vi "QueryServer_Start.vi"(7 "error in (no error)":errorcluster, 8 "Server Key File (.key)":path, 9 "Server Certificate File (.crt)":path, 10 "Server Address":string) -> (0 "error out":errorcluster, 2 "Event Registration Refnum":refnum<event-registration>, 3 "Server Info":T2)   [LabVIEW 2019, in "labview-grpc-query-server.lvlib"]
uses:
  labview-grpc-query-server.lvlib
  QueryServer_InvokeEventData.ctl
  gRPC interface/Server API/typeDefs/grpcId.ctl
  gRPC interface/Server API/typeDefs/Message Metadata.ctl
  gRPC interface/Server API/typeDefs/Message Element Metadata.ctl
  gRPC interface/Server API/typeDefs/Message Element Type.ctl
  gRPC interface/gprc-lvsupport.lvlib
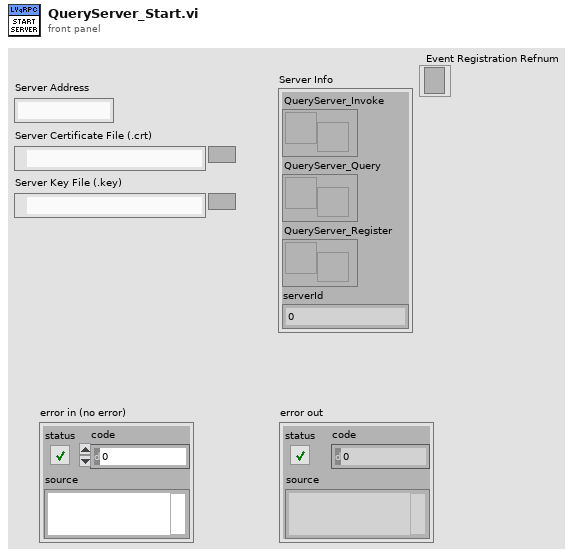
[diagram p1: front panel]
types:
  T1 = typedef "gprc-lvsupport.lvlib/grpcId.ctl" = u64
  T2 = cluster{"QueryServer_Invoke":refnum<user-event>, "QueryServer_Query":refnum<user-event>, "QueryServer_Register":refnum<user-event>, "serverId":T1}
  T3 = typedef "gprc-lvsupport.lvlib/Message Metadata.ctl" = cluster{"Name":string, "Elements":T4[]}
  T4 = typedef "gprc-lvsupport.lvlib/Message Element Metadata.ctl" = cluster{"Embedded Message Name":string, "Protobuf Index":i32, "MessageElementType":T5, "Repeated":bool}
  T5 = typedef "gprc-lvsupport.lvlib/Message Element Type.ctl" = enum32{"Int32Value", "FloatValue", "DoubleValue", "BoolValue", "StringValue", "MessageValue", ""}
  T6 = cluster{"QueryServer_Invoke":refnum<user-event>, "QueryServer_Query":refnum<user-event>, "QueryServer_Register":refnum<user-event>, "gRPCid":T1}
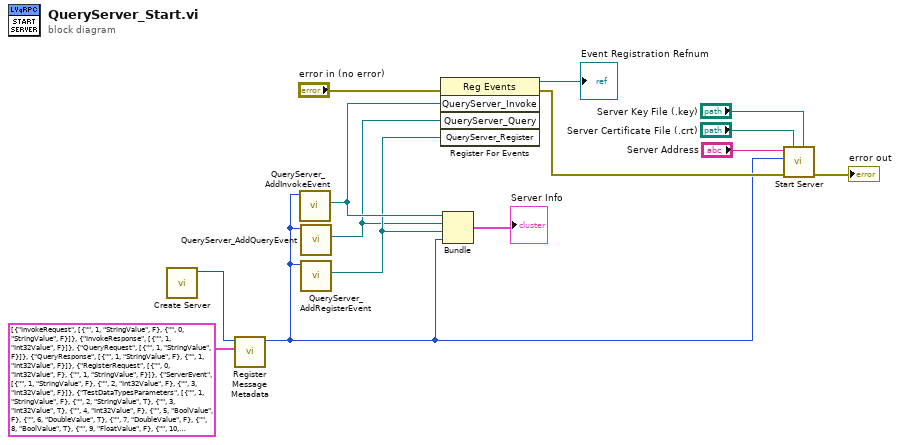
[diagram p0: block diagram]
diagram:
  n1 = call "Create Server.vi"() -> ("gRPCid"=w10:T1)  [unwired: 11 in]
  n2 = call "Register Message Metadata.vi"("Messages"=T3[] [{"Name"="InvokeRequest", "Elements"=[{"Embedded Message Name"="", "Protobuf Index"=1, "MessageElementType"=enum."StringValue", "Repeated"=FALSE}, {"Embedded Message Name"="", "Protobuf Index"=0, "MessageElementType"=enum."StringValue", "Repeated"=FALSE}]}, {"Name"="InvokeResponse", "Elements"=[{"Embedded Message Name"="", "Protobuf Index"=1, "MessageElementType"=enum."Int32Value", "Repeated"=FALSE}]}, {"Name"="QueryRequest", "Elements"=[{"Embedded Message Name"="", "Protobuf Index"=1, "MessageElementType"=enum."StringValue", "Repeated"=FALSE}]}, {"Name"="QueryResponse", "Elements"=[{"Embedded Message Name"="", "Protobuf Index"=1, "MessageElementType"=enum."StringValue", "Repeated"=FALSE}, {"Embedded Message Name"="", "Protobuf Index"=1, "MessageElementType"=enum."Int32Value", "Repeated"=FALSE}]}, {"Name"="RegisterRequest", "Elements"=[{"Embedded Message Name"="", "Protobuf Index"=0, "MessageElementType"=enum."Int32Value", "Repeated"=FALSE}, {"Embedded Message Name"="", "Protobuf Index"=1, "MessageElementType"=enum."StringValue", "Repeated"=FALSE}]}, {"Name"="ServerEvent", "Elements"=[{"Embedded Message Name"="", "Protobuf Index"=1, "MessageElementType"=enum."StringValue", "Repeated"=FALSE}, {"Embedded Message Name"="", "Protobuf Index"=2, "MessageElementType"=enum."Int32Value", "Repeated"=FALSE}, {"Embedded Message Name"="", "Protobuf Index"=3, "MessageElementType"=enum."Int32Value", "Repeated"=FALSE}]}, {"Name"="TestDataTypesParameters", "Elements"=[{"Embedded Message Name"="", "Protobuf Index"=1, "MessageElementType"=enum."StringValue", "Repeated"=FALSE}, {"Embedded Message Name"="", "Protobuf Index"=2, "MessageElementType"=enum."StringValue", "Repeated"=TRUE}, {"Embedded Message Name"="", "Protobuf Index"=3, "MessageElementType"=enum."Int32Value", "Repeated"=TRUE}, {"Embedded Message Name"="", "Protobuf Index"=4, "MessageElementType"=enum."Int32Value", "Repeated"=FALSE}, {"Embedded Message Name"="", "Protobuf Index"=5, "MessageElementType"=enum."BoolValue", "Repeated"=FALSE}, {"Embedded Message Name"="", "Protobuf Index"=6, "MessageElementType"=enum."DoubleValue", "Repeated"=TRUE}, {"Embedded Message Name"="", "Protobuf Index"=7, "MessageElementType"=enum."DoubleValue", "Repeated"=FALSE}, {"Embedded Message Name"="", "Protobuf Index"=8, "MessageElementType"=enum."BoolValue", "Repeated"=TRUE}, {"Embedded Message Name"="", "Protobuf Index"=9, "MessageElementType"=enum."FloatValue", "Repeated"=FALSE}, {"Embedded Message Name"="", "Protobuf Index"=10, "MessageElementType"=enum."FloatValue", "Repeated"=TRUE}, {"Embedded Message Name"="DataTypeTest", "Protobuf Index"=11, "MessageElementType"=enum."MessageValue", "Repeated"=FALSE}, {"Embedded Message Name"="DataTypeTest", "Protobuf Index"=12, "MessageElementType"=enum."MessageValue", "Repeated"=TRUE}]}, {"Name"="DataTypeTest", "Elements"=[{"Embedded Message Name"="", "Protobuf Index"=1, "MessageElementType"=enum."BoolValue", "Repeated"=FALSE}, {"Embedded Message Name"="", "Protobuf Index"=2, "MessageElementType"=enum."Int32Value", "Repeated"=FALSE}, {"Embedded Message Name"="", "Protobuf Index"=3, "MessageElementType"=enum."FloatValue", "Repeated"=FALSE}, {"Embedded Message Name"="", "Protobuf Index"=4, "MessageElementType"=enum."DoubleValue", "Repeated"=FALSE}]}], "gRPCid"=w10) -> ("gRPCid"=w3:T1)  [unwired: 8 in, 1 out]
  n3 = call "QueryServer_AddInvokeEvent.vi"("gRPCid in"=w3) -> ("QueryServer_Invoke"=w13:refnum<user-event>)  [unwired: 9 in, 1 out]
  n4 = call "QueryServer_AddQueryEvent.vi"("gRPCid in"=w3) -> ("QueryServer_Query"=w11:refnum<user-event>)  [unwired: 9 in, 1 out]
  n5 = call "QueryServer_AddRegisterEvent.vi"("gRPCid in"=w3) -> ("QueryServer_Register"=w12:refnum<user-event>)  [unwired: 9 in, 1 out]
  n6 = register-events(error in="error in (no error)", w13, w11, w12) -> (reference out=→"Event Registration Refnum":refnum<event-registration>, error out=w7:errorcluster)  [unwired: 1 in]
  n7 = Bundle("QueryServer_Invoke"=w13, "QueryServer_Query"=w11, "QueryServer_Register"=w12, "gRPCid"=w3) -> (→"Server Info":T6)  [unwired: 1 in]
  n8 = call "Start Server.vi"("Server Key File (.key)"="Server Key File (.key)", "Server Certificate File (.crt)"="Server Certificate File (.crt)", "error in (no error)"=w7, "gRPCid"=w3, "Server Address"="Server Address") -> ("error out"=→"error out":errorcluster)  [unwired: 6 in]
